vi "XIPIN_DDS_Compiler_6_0.vi"   [LabVIEW 2017]
doc: "The Xilinx DDS Compiler LogiCORE provides Direct Digital Synthesizers (DDS) and optionally either Phase Generator or Sine/Cosine Lookup Table constituent parts as independent cores. The core features sine, cosine or quadrature outputs with 3 to 26-bit output sample precision. The core supports up to 16 channels by time-sharing the sine/cosine table which dramatically reduces the area requirement when multiple channels are needed. Phase Dithering and Taylor Series Correction options provide high dynamic range signals using minimal FPGA resources. In addition, the core has an optional phase offset capability, providing support for multiple synthesizers with precisely controlled phase differences.\n------------------------------------\n<b>Need License</b> : No\n<b>Interface</b> : AXI4-Stream"
uses:
  <vilib>/rvi/XilinxIP/XIPIN_XNode/niFpgaXIPIN.xnode
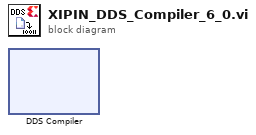
[diagram p0: block diagram]
diagram:
  n1 = xnode ("DDS Compiler")() -> ()
